vi "ReadConfigFile.vi"(8 "error in (no error)":errorcluster, 11 "MFActor in":refnum<class "MFActor.lvclass">) -> (0 "error out":errorcluster, 3 "MFActor out":refnum<class "MFActor.lvclass">)   [LabVIEW 2024, in "MFActor.lvlib" / "MFActor.lvclass"]
uses:
  MFActor.lvclass
  <vilib>/Utility/sysdir.llb/System Directory Type.ctl
  MFActor.lvclass/MFActor.ctl
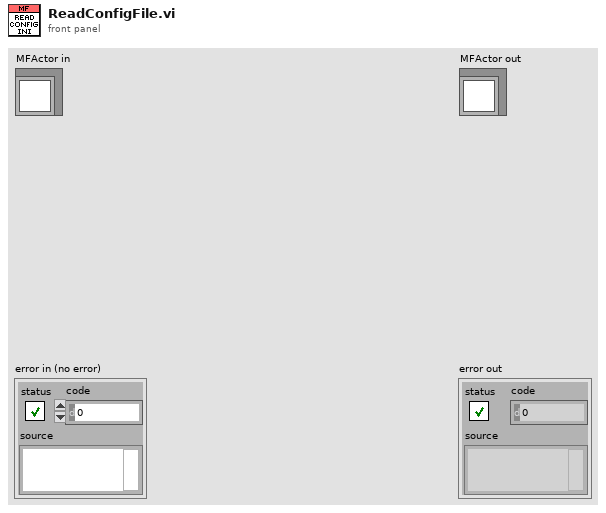
[diagram p1: front panel]
types:
  T1 = typedef "System Directory Type.ctl" = i32
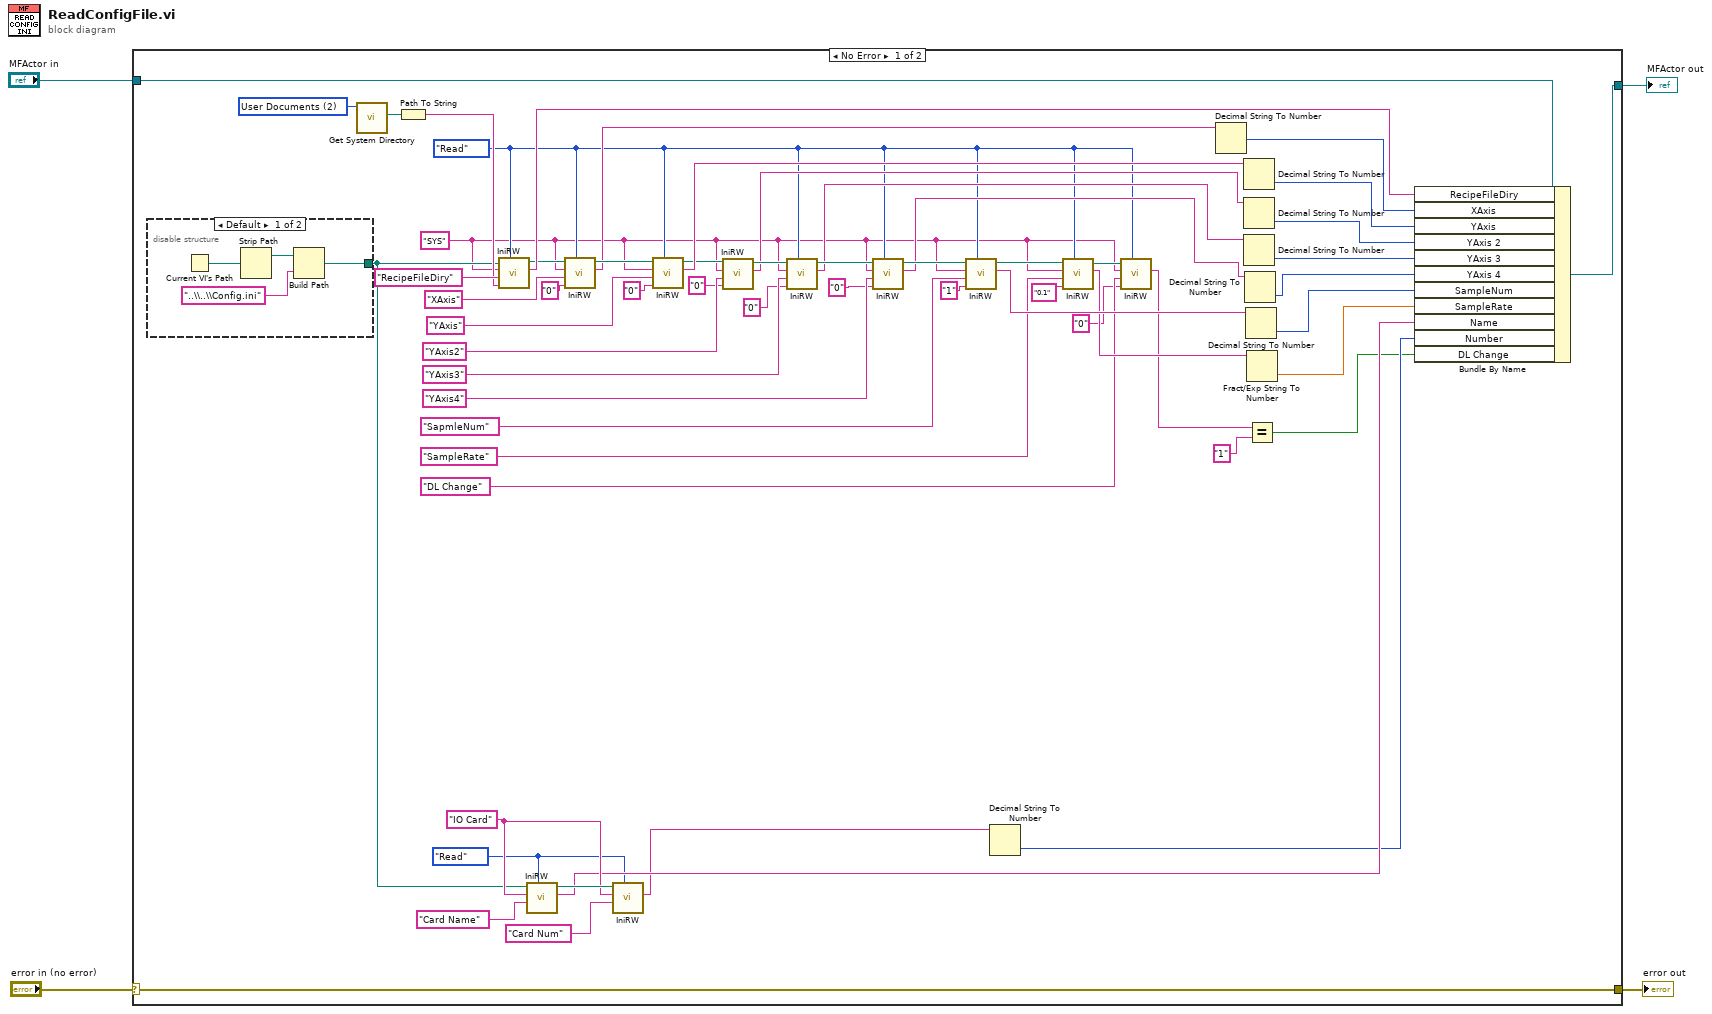
[diagram p0: block diagram]
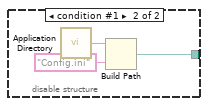
[diagram p2: hidden frame]
diagram:
  n1 = case shown="No Error" "error in (no error)" {
    selector: "error in (no error)" -> [w64 w73]
    tunnel: [w64 w73] -> w3
    tunnel: [w55 w72] -> w1
    tunnel: "MFActor in" -> [w59 w72]
    frame No Error {
      w47 = enum16{"None", "Read", "Write"}."Read" ("Operation")
      w11 = enum16{"None", "Read", "Write"}."Read" ("Operation")
      w54 = T1 2 items=["User Home"=0, "User Desktop"=1, "User Documents"=2, "User Application Data"=3, "User Preferences"=4, "User Temporary"=5, "Public Documents"=6, "Public Application Data"=7, "Public Preferences"=8, "Public Cache"=13, "System Core Libraries"=9, "System Installed Libraries"=10, "Application Files"=11, "Boot Volume Root"=12] ("system directory type")
      w10 = "SYS"
      w61 = "IO Card"
      n2 = disable-structure shown="Default" {
        disable-tunnel: [w65 w69] -> w50
        frame condition #0 (active) {
          n3 = Current VI's Path() -> (path=w68:path)
          n4 = Strip Path(path=w68) -> (stripped path=w67:path)  [unwired: 1 out]
          n5 = Build Path(base path=w67, name or relative path="..\\..\\Config.ini") -> (appended path=w65:path)
        }
        frame condition #1 {
          n6 = call <vilib>:"Application Directory.vi"() -> ("Application Directory"=w71:path)
          n7 = Build Path(base path=w71, name or relative path="Config.ini") -> (appended path=w69:path)
        }
      }
      n8 = call <vilib>:"Get System Directory.vi"("system directory type"=w54) -> ("system directory"=w52:path)  [unwired: 10 in]
      n9 = Path To String(path=w52) -> (string=w51:string)
      n10 = call "IniRW.vi"("Operation"=w11, "InputValue"=w51, "Key"="RecipeFileDiry", "Section"=w10, "IniFilePath"=w50) -> ("OutputValue"=w49:string, "IniFilePath out"=w48:path)  [unwired: 4 in, 1 out]
      n11 = call "IniRW.vi"("Operation"=w47, "Key"="Card Name", "Section"=w61, "IniFilePath"=w50) -> ("OutputValue"=w58:string, "IniFilePath out"=w62:path)  [unwired: 5 in, 1 out]
      n12 = call "IniRW.vi"("Operation"=w11, "InputValue"="0", "Key"="XAxis", "Section"=w10, "IniFilePath"=w48) -> ("OutputValue"=w41:string, "IniFilePath out"=w44:path)  [unwired: 4 in, 1 out]
      n13 = call "IniRW.vi"("Operation"=w47, "Key"="Card Num", "Section"=w61, "IniFilePath"=w62) -> ("OutputValue"=w57:string)  [unwired: 5 in, 2 out]
      n14 = call "IniRW.vi"("Operation"=w11, "InputValue"="0", "Key"="YAxis", "Section"=w10, "IniFilePath"=w44) -> ("OutputValue"=w39:string, "IniFilePath out"=w29:path)  [unwired: 4 in, 1 out]
      n15 = call "IniRW.vi"("InputValue"="0", "Key"="YAxis2", "Section"=w10, "IniFilePath"=w29) -> ("OutputValue"=w19:string, "IniFilePath out"=w28:path)  [unwired: 5 in, 1 out]
      n16 = call "IniRW.vi"("Operation"=w11, "InputValue"="0", "Key"="YAxis3", "Section"=w10, "IniFilePath"=w28) -> ("OutputValue"=w18:string, "IniFilePath out"=w27:path)  [unwired: 4 in, 1 out]
      n17 = call "IniRW.vi"("Operation"=w11, "InputValue"="0", "Key"="YAxis4", "Section"=w10, "IniFilePath"=w27) -> ("OutputValue"=w16:string, "IniFilePath out"=w17:path)  [unwired: 4 in, 1 out]
      n18 = call "IniRW.vi"("Operation"=w11, "InputValue"="1", "Key"="SapmleNum", "Section"=w10, "IniFilePath"=w17) -> ("OutputValue"=w36:string, "IniFilePath out"=w34:path)  [unwired: 4 in, 1 out]
      n19 = Decimal String To Number(string=w57) -> (number=w56:i32)  [unwired: 2 in, 1 out]
      n20 = call "IniRW.vi"("Operation"=w11, "InputValue"="0.1", "Key"="SampleRate", "Section"=w10, "IniFilePath"=w34) -> ("OutputValue"=w31:string, "IniFilePath out"=w12:path)  [unwired: 4 in, 1 out]
      n21 = call "IniRW.vi"("Operation"=w11, "InputValue"="0", "Key"="DL Change", "Section"=w10, "IniFilePath"=w12) -> ("OutputValue"=w6:string)  [unwired: 4 in, 2 out]
      n22 = Decimal String To Number(string=w41) -> (number=w40:i32)  [unwired: 2 in, 1 out]
      n23 = Decimal String To Number(string=w39) -> (number=w20:i32)  [unwired: 2 in, 1 out]
      n24 = Decimal String To Number(string=w19) -> (number=w15:i32)  [unwired: 2 in, 1 out]
      n25 = Decimal String To Number(string=w18) -> (number=w14:i32)  [unwired: 2 in, 1 out]
      n26 = Decimal String To Number(string=w16) -> (number=w13:i32)  [unwired: 2 in, 1 out]
      n27 = Decimal String To Number(string=w36) -> (number=w35:i32)  [unwired: 2 in, 1 out]
      n28 = Fract/Exp String To Number(string=w31) -> (number=w30:dbl)  [unwired: 3 in, 1 out]
      n29 = Equal?(x=w6, y="1") -> (x = y?=w5:bool)
      n30 = Bundle By Name(cluster=w59, "RecipeFileDiry"=w49, "XAxis"=w40, "YAxis"=w20, "YAxis 2"=w15, "YAxis 3"=w14, "YAxis 4"=w13, "SampleNum"=w35, "SampleRate"=w30, "Name"=w58, "Number"=w56, "DL Change"=w5) -> (w55:refnum<class "MFActor.lvclass">)
    }
    frame Error {
    }
  }
  "error out" <- w3
  "MFActor out" <- w1
